vi "SetChangeTaskSampleTrigger.vi"(0 "controller in":refnum<k24>, 5 "signal":i32(ring)=17 items=["ProgramLineNumber"=17, "CoordinatedFlags"=45, "CoordinatedArcStartAngle"=58, "CoordinatedArcEndAngle"=59, "CoordinatedArcRadius"=60, "CoordinatedArcRadiusError"=61, "CoordinatedPositionCommand"=62, "CoordinatedSpeedCommand"=63, "CoordinatedAccelerationCommand"=64, "CoordinatedTotalDistance"=65, "CoordinatedPercentDone"=66, "CoordinatedPositionCommandBackwardsDiff"=67, "ProgramVariable"=75, "TaskParameter"=77, "TaskErrorCode"=79, "TaskWarningCode"=80, "DwellCommandPercentComplete"=102, "WaitCommandDuration"=103, "CoordinatedSpeedTargetActual"=104, "DependentCoordinatedSpeedTargetActual"=105, "ActiveFixtureOffset"=106, "TaskStatus0"=108, "TaskStatus1"=109, "TaskStatus2"=110, "ProgramLineNumberNoSync"=111, "Spindle0SpeedTarget"=112, "Spindle1SpeedTarget"=113, "Spindle2SpeedTarget"=114, "Spindle3SpeedTarget"=115, "CoordinateSystem1I"=118, "CoordinateSystem1J"=119, "CoordinateSystem1K"=120, "CoordinateSystem1Plane"=121, "ToolNumberActive"=122, "MFO"=123, "CoordinatedSpeedTarget"=124, "DependentCoordinatedSpeedTarget"=125, "CoordinatedAccelerationRate"=132, "CoordinatedDecelerationRate"=133, "CoordinatedAccelerationTime"=134, "CoordinatedDecelerationTime"=135, "TaskMode"=137, "TaskState"=146, "TaskStateInternal"=147, "ExecutionMode"=151, "TaskErrorLocation"=152, "TaskWarningLocation"=153, "ProgramPersistent"=154, "ImmediateState"=155, "EnableAlignmentAxes"=159, "QueueStatus"=162, "CoordinatedGalvoLaserOutput"=169, "CoordinatedMotionRate"=184, "CoordinatedTaskCommand"=185, "FiberMoveCount"=195, "EnableState"=224, "CannedFunctionID"=240, "TaskDoubleVariable"=248, "TaskInfoVariable"=249, "TaskReturnVariable"=271, "FiberPower"=273, "FiberPowerOptimal"=274, "FiberPowerSampleCount"=275, "FiberSearchResult"=276, "LookaheadMovesExamined"=278, "LookaheadMovesRecomputed"=279, "ProgramLineNumberInternal"=322, "ProfileControlMask"=324, "QueueLineCount"=325, "QueueLineCapacity"=326, "ImmediateCommandErrorCode"=329, "ImmediateCommandErrorLocation"=330, "LookaheadErrorCode"=335, "LookaheadErrorLocation"=336, "LookaheadMovePoolIndex"=337, "ActiveMovePoolIndex"=338, "CoordinatedArcRadiusReciprocal"=363, "ActiveMoveElementAddedOrderIndex"=364, "MotionEngineStage"=367, "CoordinatedTimeScale"=370, "CoordinatedTimeScaleDerivative"=371, "IFOVTimeScale"=380, "IFOVTimeScaleAverage"=381, "IFOVGenerationFrameCounter"=382, "IFOVGenerationTimeOriginal"=383, "IFOVGenerationTimeModified"=384, "IFOVCoordinatedPositionCommand"=385, "IFOVCoordinatedSpeedCommand"=386, "IFOVCenterPointH"=390, "IFOVCenterPointV"=391, "IFOVTrajectoryCount"=392, "IFOVTrajectoryIndex"=393, "IFOVAttemptCode"=394, "IFOVGenerationFrameIndex"=395, "IFOVMaximumVelocity"=396, "IFOVIdealVelocity"=397, "TaskInternalDebug"=398, "IFOVCoordinatedAccelerationCommand"=399, "IFOVFOVPositionH"=400, "IFOVFOVPositionV"=401, "IFOVFOVDimensionH"=402, "IFOVFOVDimensionV"=403, "CoordinatedTimeSkipped"=406], 7 "task":i32, 9 "optional":i32, 11 "error in (no error)":errorcluster, 12 "trigger":i32(ring)=1 items=["OnAnyChange"=1, "OnIncrease"=2, "OnDecrease"=3]) -> (4 "controller out":refnum<k24>, 15 "error out":errorcluster)   [LabVIEW 2016, in "Aerotech VIs.lvlib"]
uses:
  Aerotech VIs.lvlib
  C:/Program Files (x86)/Aerotech/A3200/LabVIEW/2010/Bin/Aerotech.A3200.dll
  C:/Program Files (x86)/Aerotech/A3200/LabVIEW/2010/Bin/Aerotech.A3200.LabVIEW.dll
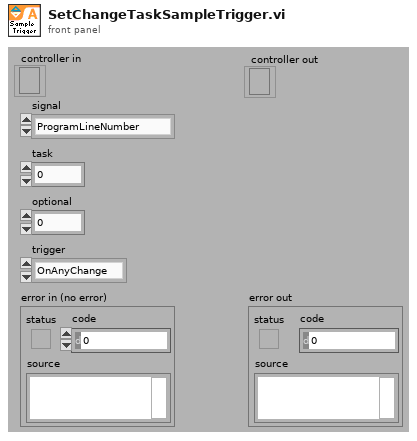
[diagram p1: front panel]
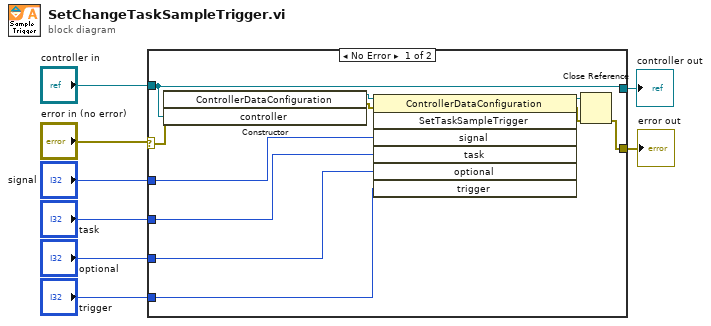
[diagram p0: block diagram]
diagram:
  n1 = case shown="No Error" "error in (no error)" {
    selector: "error in (no error)" -> [w19 w21]
    tunnel: "controller in" -> [w14 w20]
    tunnel: [w11 w21] -> w5
    tunnel: [w14 w20] -> w6
    tunnel: "optional" -> [w15 _]
    tunnel: "trigger" -> [w16 _]
    tunnel: "task" -> [w10 _]
    tunnel: "signal" -> [w9 _]
    frame No Error {
      n2 = constructor class="ControllerDataConfiguration"(error in=w19, "controller"=w14) -> (reference out=w18:refnum<k24>, error out=w17:errorcluster)  [unwired: 2 in, 2 out]
      n3 = invoke class="ControllerDataConfiguration" method="SetTaskSampleTrigger"(reference=w18, error in=w17, "signal"=w9, "task"=w10, "optional"=w15, "trigger"=w16) -> (reference out=w12:refnum<k24>, error out=w13:errorcluster)  [unwired: 1 in, 5 out]
      n4 = Close Reference(reference=w12, error in (no error)=w13) -> (error out=w11:errorcluster)
    }
    frame Error {
    }
  }
  "controller out" <- w6
  "error out" <- w5
